vi "SUB_ASKLEDSBlinking_AllOn.vi"() -> (1 "NewVal":T1(ring))   [LabVIEW 2011]
doc: "This is an example of how to use the radio buttons control with the Value Changed event."
panel:
  out "yes/no":T2(ring)=enum."None"
  in  "Answer Question(如上述所述, 為Pass,否則為NG)":T1(radio)=enum."Yes"
  # "右下4顆LED是依序燈亮 至滅(不亮)"
  # "重測"
  # "NG"
  # "PASS"
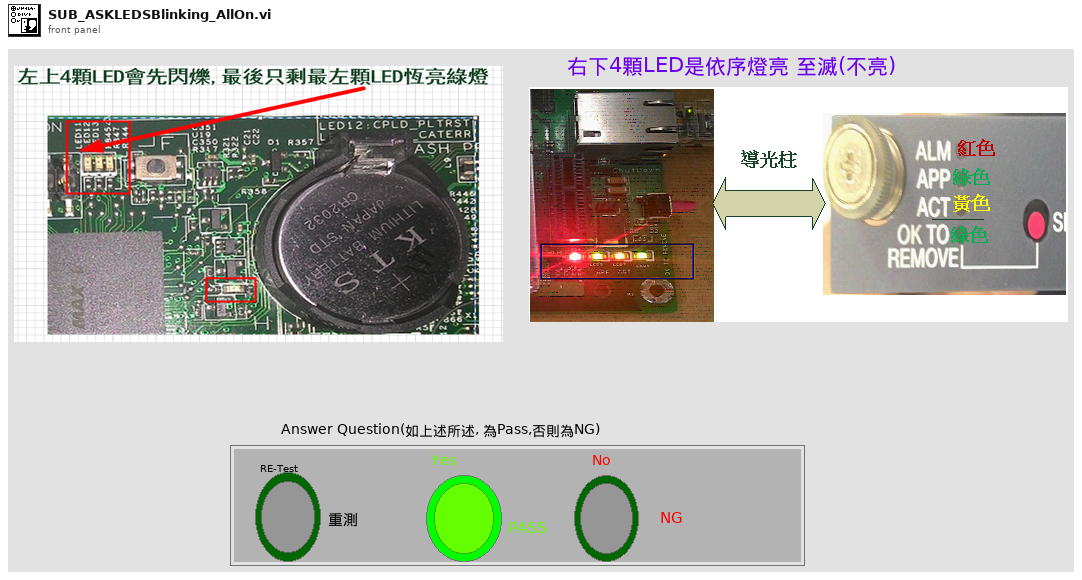
[diagram p1: front panel]
types:
  T1 = enum32{"No Selection", "Yes", "No", "None", "RE-Test"}
  T2 = enum32{"No Selection", "Yes", "No", "None", "Retest"}
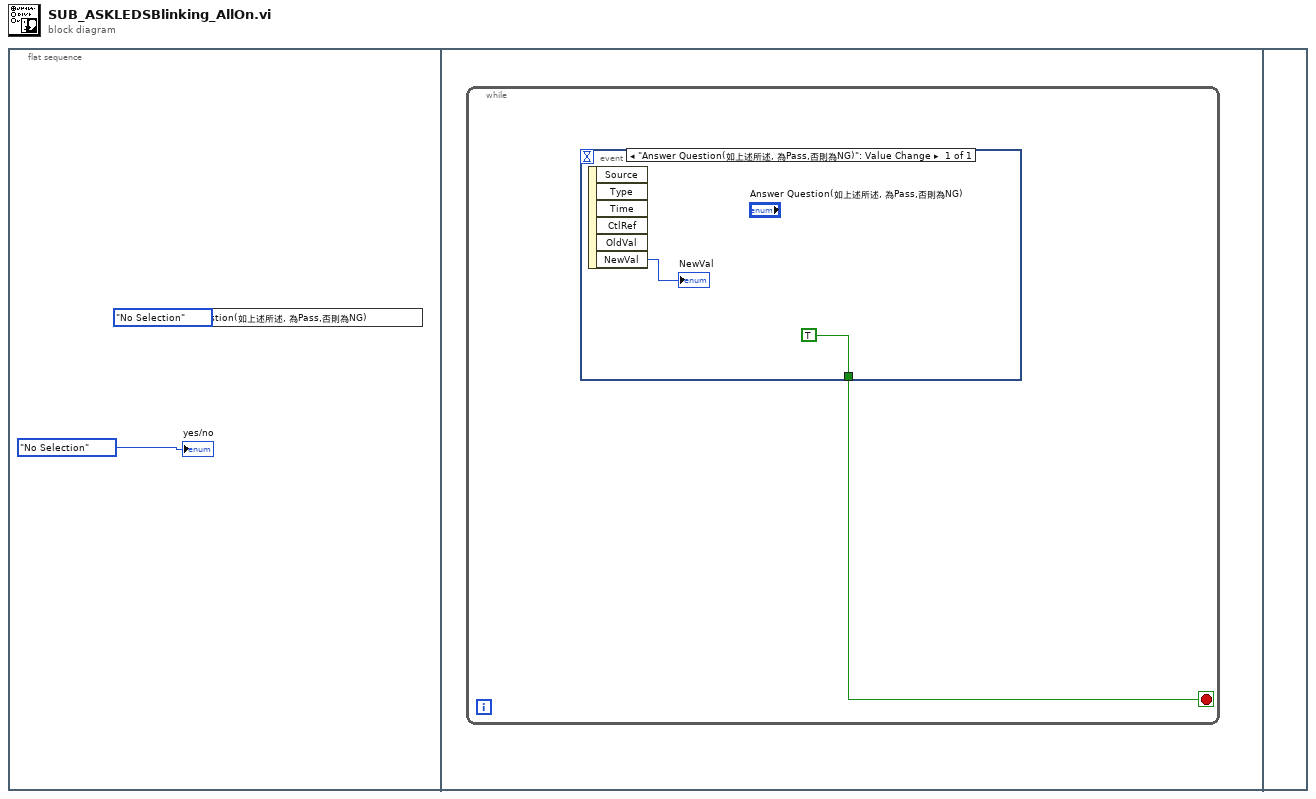
[diagram p0: block diagram]
diagram:
  n1 = flat-sequence {
    frame #0 {
      n2 = local write "Answer Question(如上述所述, 為Pass,否則為NG)"(T1."No Selection" ("Answer Question")) -> ()
      "yes/no" <- T2."No Selection" ("yes/no")
    }
    frame #1 {
      n3 = while {
        stop <- w3 stop-if-true
        n4 = event shown="[0] \"Answer Question(如上述所述, 為Pass,否則為NG)\": Value Change" {
          selector: _ -> [_]
          dyn-events: _ -> [_]
          timeout: _ -> [_]
          tunnel: [TRUE] -> w3
          event "Answer Question(如上述所述, 為Pass,否則為NG)": Value Change {
            n5 = event-data() -> ("NewVal"=→"NewVal":T1)  [unwired: 1 in, 5 out]
          }
        }
      }
    }
    frame #2 {
    }
  }
